vi "Read dt (s).vi"(11 "PID Timing Estimation in":refnum<class "PID Timing Estimation.lvclass">) -> (2 "dt (s)":dbl, 3 "PID Timing Estimation out":refnum<class "PID Timing Estimation.lvclass">)   [LabVIEW 2019, in "control.lvlib" / "PID Timing Estimation.lvclass"]
uses:
  PID Timing Estimation.lvclass
  PID Timing Estimation.lvclass/PID Timing Estimation.ctl
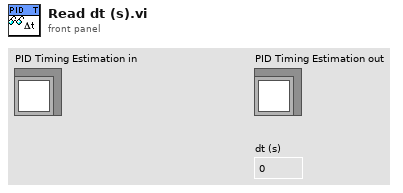
[diagram p1: front panel]
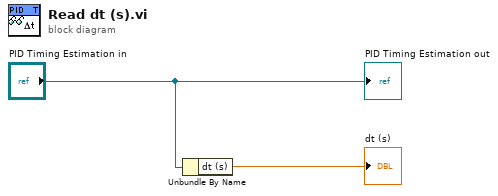
[diagram p0: block diagram]
diagram:
  n1 = Unbundle By Name("PID Timing Estimation in") -> ("dt (s)"=→"dt (s)":dbl)
  "PID Timing Estimation out" <- "PID Timing Estimation in"
